vi "机械手DEMO.vi"() -> ()   [LabVIEW 2013]
uses:
  <vilib>/Statechart/Common/IntGuid.ctl
  <vilib>/Statechart/Common/DbgID.ctl
  <vilib>/Statechart/Infrastructure/RTStatechart/RunTime SCN.xnode
  <vilib>/Statechart/Common/NI_SC_LVSCCommonFiles.lvlib
panel:
  out "Outputs":T1
  in  "Inputs":T2
  in  "停止":bool
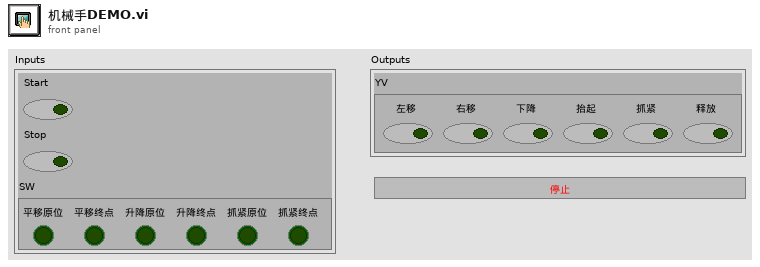
[diagram p1: front panel]
types:
  T1 = typedef "机械手.lvsc/Outputs.ctl" = cluster{"YV":cluster{"左移":bool, "右移":bool, "下降":bool, "抬起":bool, "抓紧":bool, "释放":bool}}
  T2 = typedef "机械手.lvsc/Inputs.ctl" = cluster{"Start":bool, "Stop":bool, "SW":cluster{"平移原位":bool, "平移终点":bool, "升降原位":bool, "升降终点":bool, "抓紧原位":bool, "抓紧终点":bool}}
  T3 = typedef "机械手.lvsc/Trigger.ctl" = enum16{"NULL"}
  T4 = typedef "NI_SC_LVSCCommonFiles.lvlib/IntGuid.ctl" = cluster{"Data1":u32, "Data2":u16, "Data3":u16, "Data4":u8, "Data5":u8, "Data6":u8, "Data11":u8, "Data9":u8, "Data10":u8, "Data8":u8, "Data7":u8}
  T5 = typedef "NI_SC_LVSCCommonFiles.lvlib/DbgID.ctl" = cluster{"VIRef":u32, "IntGUID":T4}
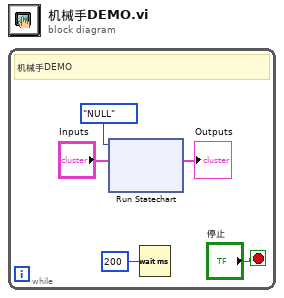
[diagram p0: block diagram]
diagram:
  n1 = while {
    stop <- "停止" stop-if-true
    # "机械手DEMO"
    n2 = xnode "Run Statechart"("Inputs"="Inputs", "Trigger"=Trigger."NULL") -> ("Outputs"=→"Outputs":T1)  [unwired: 1 in, 1 out]
    n3 = Wait (ms)(milliseconds to wait=u32 200 ("等待时间（毫秒）")) -> ()  [unwired: 1 out]
  }
